vi "poly_lock_fp_updates_unlock_vi_ref.vi"(8 "error in":errorcluster, 9 "vi ref":refnum<vi>) -> (0 "error out":errorcluster)   [LabVIEW 2015]
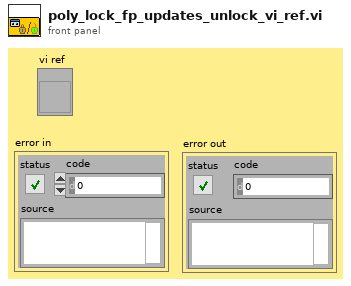
[diagram p1: front panel]
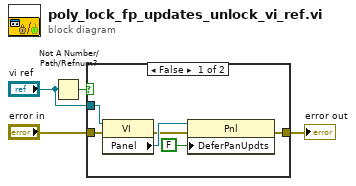
[diagram p0: block diagram]
diagram:
  n1 = Not A Number/Path/Refnum?(number/path/refnum="vi ref") -> (NaN/Path/Refnum?=w2:bool)
  n2 = case shown="False" w2 {
    tunnel: [w9 w11] -> w4
    tunnel: "error in" -> [w5 w11]
    tunnel: "vi ref" -> [w8 _]
    frame False {
      n3 = property class="VI"(reference=w8, error in=w5) -> (error out=w6:errorcluster, "Panel"=w7:refnum<vi>)  [unwired: 1 out]
      n4 = property class="Pnl"(reference=w7, error in=w6, "DeferPanUpdts"=FALSE) -> (error out=w9:errorcluster)  [unwired: 1 out]
    }
    frame True {
    }
  }
  "error out" <- w4
